vi "counter_test.vi"() -> ()   [LabVIEW 2009]
panel:
  out "x/y":i16
  out "output array":i16[](array[numeric])
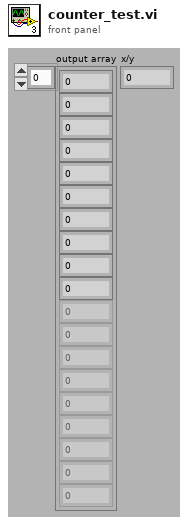
[diagram p1: front panel]
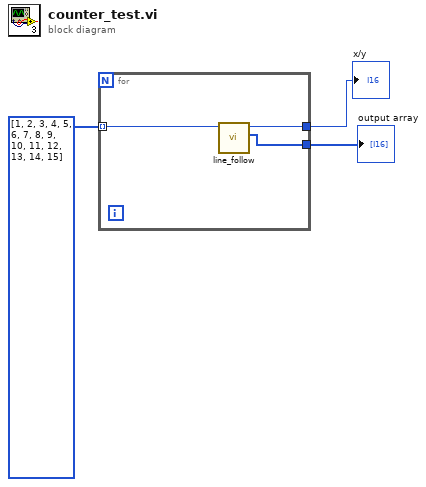
[diagram p0: block diagram]
diagram:
  n1 = for {
    tunnel: i16[] [1, 2, 3, 4, 5, 6, 7, 8, 9, 10, 11, 12, 13, 14, 15] -> [w6] mode=indexing
    tunnel: [w5] -> w2
    tunnel: [w4] -> w1
    n2 = call "line_follow.vi"("New Heading"=w6) -> ("output array"=w5:i16[], "x/y"=w4:i16)  [unwired: 9 in]
  }
  "output array" <- w2
  "x/y" <- w1
